vi "Fat16 timestamp calc.vi"(10 "time stamp":timestamp) -> (2 "timestamp as string":string)   [LabVIEW 2014]
panel:
  out "timestamp as int":i32 format="%8x"
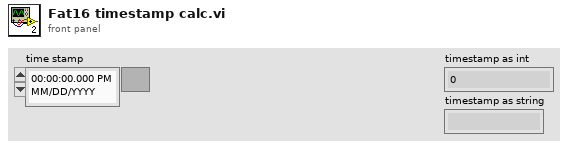
[diagram p1: front panel]
types:
  T1 = typedef "LVDateTimeRec.ctl" = cluster{"fractional second":dbl, "second":i32, "minute":i32, "hour":i32, "day of month":i32, "month":i32, "year":i32, "day of week":i32, "day of year":i32, "DST":i32}
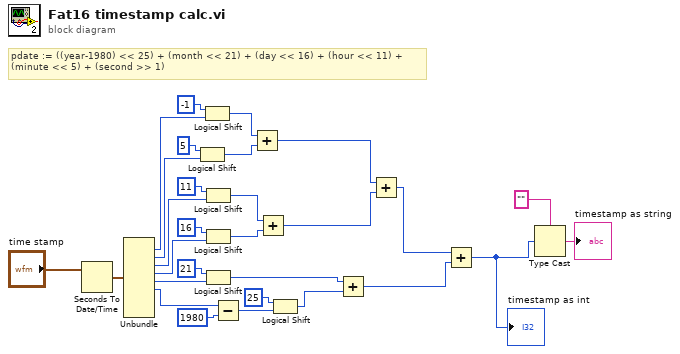
[diagram p0: block diagram]
diagram:
  # "pdate := ((year-1980) << 25) + (month << 21) + (day << 16) + (hour << 11) + (minute << 5) + (second >> 1)"
  n1 = Seconds To Date/Time(time stamp (now)="time stamp") -> (date time rec=w29:T1)  [unwired: 1 in]
  n2 = Unbundle(w29) -> ("second"=w18:i32, "minute"=w17:i32, "hour"=w16:i32, "day of month"=w15:i32, "month"=w14:i32, "year"=w27:i32)  [unwired: 4 out]
  n3 = Logical Shift(y=i16 5, x=w17) -> (x << y=w13:i32)
  n4 = Logical Shift(y=i16 -1, x=w18) -> (x << y=w12:i32)
  n5 = Logical Shift(y=i16 11, x=w16) -> (x << y=w8:i32)
  n6 = Logical Shift(y=i16 16, x=w15) -> (x << y=w9:i32)
  n7 = Logical Shift(y=i16 21, x=w14) -> (x << y=w10:i32)
  n8 = Subtract(x=w27, y=1980) -> (x-y=w25:i32)
  n9 = Add(x=w12, y=w13) -> (x+y=w4:i32)
  n10 = Add(x=w8, y=w9) -> (x+y=w7:i32)
  n11 = Logical Shift(y=i16 25, x=w25) -> (x << y=w11:i32)
  n12 = Add(x=w10, y=w11) -> (x+y=w5:i32)
  n13 = Add(x=w4, y=w7) -> (x+y=w6:i32)
  n14 = Add(x=w6, y=w5) -> (x+y=w3:i32)
  "timestamp as int" <- w3
  n15 = Type Cast(type="", x=w3) -> (*(type *) &x=→"timestamp as string":string)
